vi "get first and last index.vi"(11 "Channels In":T1[](array[typedef]) {"Mapping"."VS Reference" format="%.0x"}) -> (1 "length":u16, 2 "Last Register":i32, 3 "Starting Register":u16)   [LabVIEW 2021, in "Modbus Master System Explorer.lvlib"]
uses:
  Modbus Master System Explorer.lvlib
  Shared/Controls/Data Model/Channel.ctl
  Modbus Type.ctl
  <vilib>/NI VeriStand/Custom Device API/Custom Device Channel Type.ctl
  Shared/Controls/Data Model/Mapping.ctl
  Shared/Controls/Data Model/DataType.ctl
  <vilib>/NI VeriStand/Custom Device API/Custom Device Item Ref.ctl
  Shared/Modbus Master Shared.lvlib
  <vilib>/NI VeriStand/Custom Device API/Custom Device API.lvlib
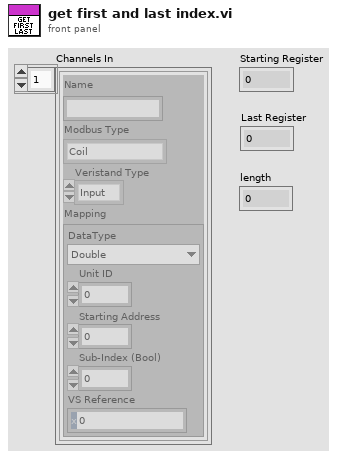
[diagram p1: front panel]
types:
  T1 = typedef "Modbus Master Shared.lvlib/Channel.ctl" = cluster{"Name":string, "Modbus Type":T2, "Veristand Type":T3, "Mapping":T4}
  T2 = typedef "Modbus Master Shared.lvlib/Modbus Type.ctl" = enum16{"Coil", "Discrete Input", "Holding Register", "Input Register"}
  T3 = typedef "Custom Device API.lvlib/Custom Device Channel Type.ctl" = enum16{"Input", "Output"}
  T4 = typedef "Modbus Master Shared.lvlib/Mapping.ctl" = cluster{"DataType":T5, "Unit ID":u8, "Starting Address":u16, "Sub-Index (Bool)":u16, "VS Reference":T6}
  T5 = typedef "Modbus Master Shared.lvlib/DataType.ctl" = enum16{"Double", "Single", "I64", "I32", "I16", "I8", "U64", "U32", "U16", "U8", "Boolean"}
  T6 = typedef "Custom Device API.lvlib/Custom Device Item Ref.ctl" = u64
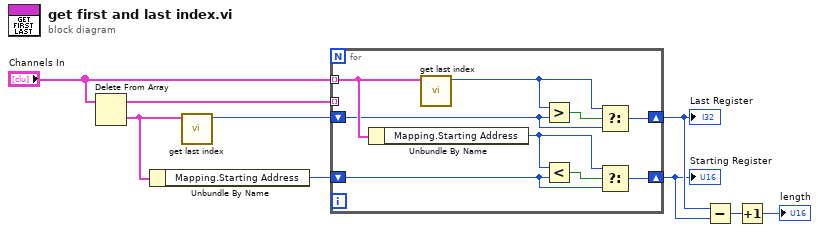
[diagram p0: block diagram]
diagram:
  n1 = Delete From Array(array="Channels In") -> (deleted portion=w7:T1, array with subset deleted=w6:T1[])  [unwired: 2 in]
  n2 = Unbundle By Name(w7) -> ("Mapping.Starting Address"=w8:u16)
  n3 = call "get last index.vi"("Channel"=w7) -> ("Last Index"=w9:u16)  [unwired: 10 in]
  n4 = for {
    tunnel: "Channels In" -> [w18] mode=indexing
    shift-right: [w14] -> w3
    shift-left: w8 -> [w15]
    tunnel: w6 -> [_] mode=indexing
    shift-right: [w10] -> w4
    shift-left: w9 -> [w11]
    n5 = Unbundle By Name(w18) -> ("Mapping.Starting Address"=w16:u16)
    n6 = call "get last index.vi"("Channel"=w18) -> ("Last Index"=w12:u16)  [unwired: 10 in]
    n7 = Greater?(x=w12, y=w11) -> (0:w13:bool)
    n8 = Less?(x=w16, y=w15) -> (x < y?=w17:bool)
    n9 = Select(t=w12, s=w13, f=w11) -> (s? t:f=w10:u16)
    n10 = Select(t=w16, s=w17, f=w15) -> (s? t:f=w14:u16)
  }
  "Starting Register" <- w3
  "Last Register" <- w4
  n11 = Subtract(x=w4, y=w3) -> (x-y=w2:u16)
  n12 = Increment(x=w2) -> (x+1=→"length":u16)
